vi "Dashboard Main.vi"() -> ()   [LabVIEW 2013]
uses:
  <vilib>/event_ctls.llb/eventvkey.ctl
  <vilib>/Rock Robotics/WPI/Dashboard/WPI_DashboardLogging Global.vi
  <vilib>/Utility/config.llb/Write Key (String).vi
  <vilib>/Utility/config.llb/Write Key (I32).vi
  <vilib>/Utility/config.llb/NI_LVConfig.lvlib
panel:
  out "Image Message":string="Timeout in Camera Communications"
  in  "Rec Mode":enum32{"Stop", "Record", "Playback"}(radio)
  in  "Dashboard Tab":T1(tab)
  in  "Camera Settings":T2={"Frame Rate"=30, "Compression"=30, "Size"=1} {"Frame Rate" scale=1.0..30.0; "Size" items=["640x480", "320x240", "160x120"]}
  out "MotorSliders R":cluster{"MotorSlide1":dbl, "MotorSlide2":dbl} {"MotorSlide2" scale=-1.0..1.0 scale format="%#_2e"; "MotorSlide1" scale=-1.0..1.0 scale format="%#_2e"}
  out "MotorChart R":cluster{"Numeric":dbl, "Numeric":dbl}(graph)
  out "MotorSliders L":T3 {"MotorSlide4 2" scale=0.0..14.0 scale format="%#_2e"; "MotorSlide2" scale=-1.0..1.0 scale format="%#_2e"; "MotorSlide1" scale=-1.0..1.0 scale format="%#_2e"}
  out "MotorChart L":T4(graph)
  out "JS1 Z":dbl(slide) scale=-1.0..1.0 scale format="%#_2e"
  out "Joystick 1":cluster{"X":dbl, "Y":dbl}[](graph)
  out "JS Buttons 1":T5
  out "JS2 Z":dbl(slide) scale=-1.0..1.0 scale format="%#_2e"
  out "Joystick 2":cluster{"X":dbl, "Y":dbl}[](graph)
  out "JS Buttons 2":T5
  out "Mode":T6(ring)=enum."Auto Disabled"
  out "Camera IP":string
  in  "DB Camera Config":bool
  out "fps":dbl format="%#.1g"
  out "Mbps":dbl format="%#.1g"
  out "Mbps 2":bool
  out "LED 1":bool
  in  "Shooter Angle":dbl(slide) scale=20.0..40.0
  out "Averaged Shooter Speed":dbl
  in  "Shooter Speed":dbl(slide) scale=0.0..9.0
  in  "Checkbox 2":bool
  in  "Checkbox 1":bool
  in  "Test Slider":dbl(slide) scale=0.0..100.0 scale format="%#_3g"
  in  "On/Off":bool caption="Solenoid"
  in  "Test Name":u16(ring) items=["Select the test to run...", "Example Test", "-------------------------------", "List of tests is built in robot code.", "Replace with your own automated tests."]
  in  "Test Tree":string(tree)
  in  "Motor":cluster{"Value":dbl, "Enable":bool} {"Value" scale=-1.0..1.0 scale format="%#_3g"}
  out "Progress":T7 {"Test Progress" scale=0.0..100.0}
  in  "Rev/Fwd":cluster{"Forward":bool, "Reverse":bool}
  in  "Test Ring":u16(ring) items=["Auto", "Fixed indoor", "Fixed outdoor 1", "Fixed outdoor 2", "Fixed fluorescent 1", "Fixed fluorescent 2", "Hold current"]
  in  "Listbox":i32(listbox)
  out "Tree":string(tree)
  out "Camera Image":T8(plugin-control)
  in  "Enable":bool
  # "Left"
  # "Front"
  # "Right"
  # "Battery"
  # "This tab is a great place for autonomous settings and validation.\nCustomize by placing controls and indicators here and name to\nmatch Dashboard Variables on robot."
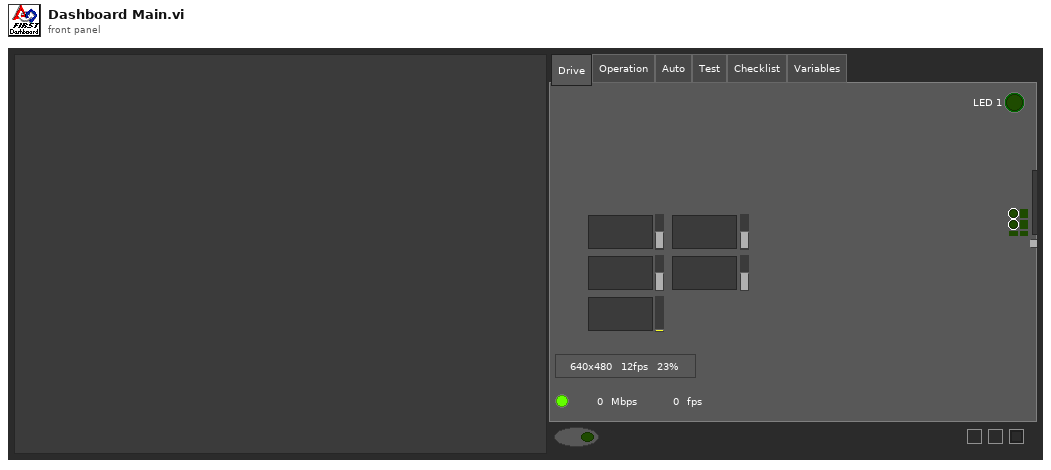
[diagram p1: front panel]
types:
  T1 = enum32{"Drive", "Operation", "Auto", "Test", "Checklist", "Variables"}
  T2 = cluster{"Frame Rate":i32, "Compression":i32, "Size":u16}
  T3 = cluster{"MotorSlide1":dbl, "MotorSlide2":dbl, "MotorSlide4 2":dbl}
  T4 = cluster{"Numeric":dbl, "Numeric":dbl, "Battery":sgl}
  T5 = cluster{bool, bool, bool, bool, bool, bool, bool, bool, bool, bool, bool, bool}
  T6 = enum8{"Tele-Op Disabled", "Tele-Op Enabled", "Auto Disabled", "Auto Enabled", "Test Disabled", "Test Enabled", ""}
  T7 = cluster{"Test Progress":u8, "Test Progress Text":string}
  T8 = typedef "IMAQ Image.ctl" = refnum<image>
  T9 = typedef "Image Type" = u32
  T10 = cluster{"Digital Inputs":bool[], "Digital Outputs":bool[]}
  T11 = cluster{"Competition mode":bool, "Robot Link":bool, "Autonomous":bool, "Enabled":bool, "E-Stop":bool, "Simulated":bool, "TestMode":bool, "Docked Window":bool}
  T12 = cluster{"Boolean Array[0]":bool, "Boolean Array[1]":bool, "Boolean Array[2]":bool, "Boolean Array[3]":bool, "Boolean Array[4]":bool, "Boolean Array[5]":bool, "Boolean Array[6]":bool, "Boolean Array[7]":bool, "Boolean Array[8]":bool, "Boolean Array[9]":bool, "Boolean Array[10]":bool, "Boolean Array[11]":bool}
  T13 = typedef "NI_LVConfig.lvlib/Config Data RefNum.ctl" = refnum<k1>
  T14 = typedef "eventvkey.ctl" = enum16{"ASCII", "Enter", "Return", "Shift", "Ctrl", "Alt", "Cmd", "Opt", "Caps", "NumLock", "Clear", "Break", "Up", "Down", "Left", "Right", "Insert", "Delete", "Home", "End", "PageUp", "PageDown", "Escape", "Help", "Pause", "ScrollLock", "F1", "F2", "F3", "F4", "F5", "F6", "F7", "F8", "F9", "F10", "F11", "F12", "F13", "F14", "F15", "F16", "F17", "F18", "F19", "F20", "F21", "F22", "F23", "F24", "Play", "VolumeUp", "VolumeDown", "Mute", "Two Byte Char"}
  T15 = cluster{"Image Size":bool, "Image Type":bool, "Pixel Value":bool, "ROI Information":bool, "Zoom Factor":bool}
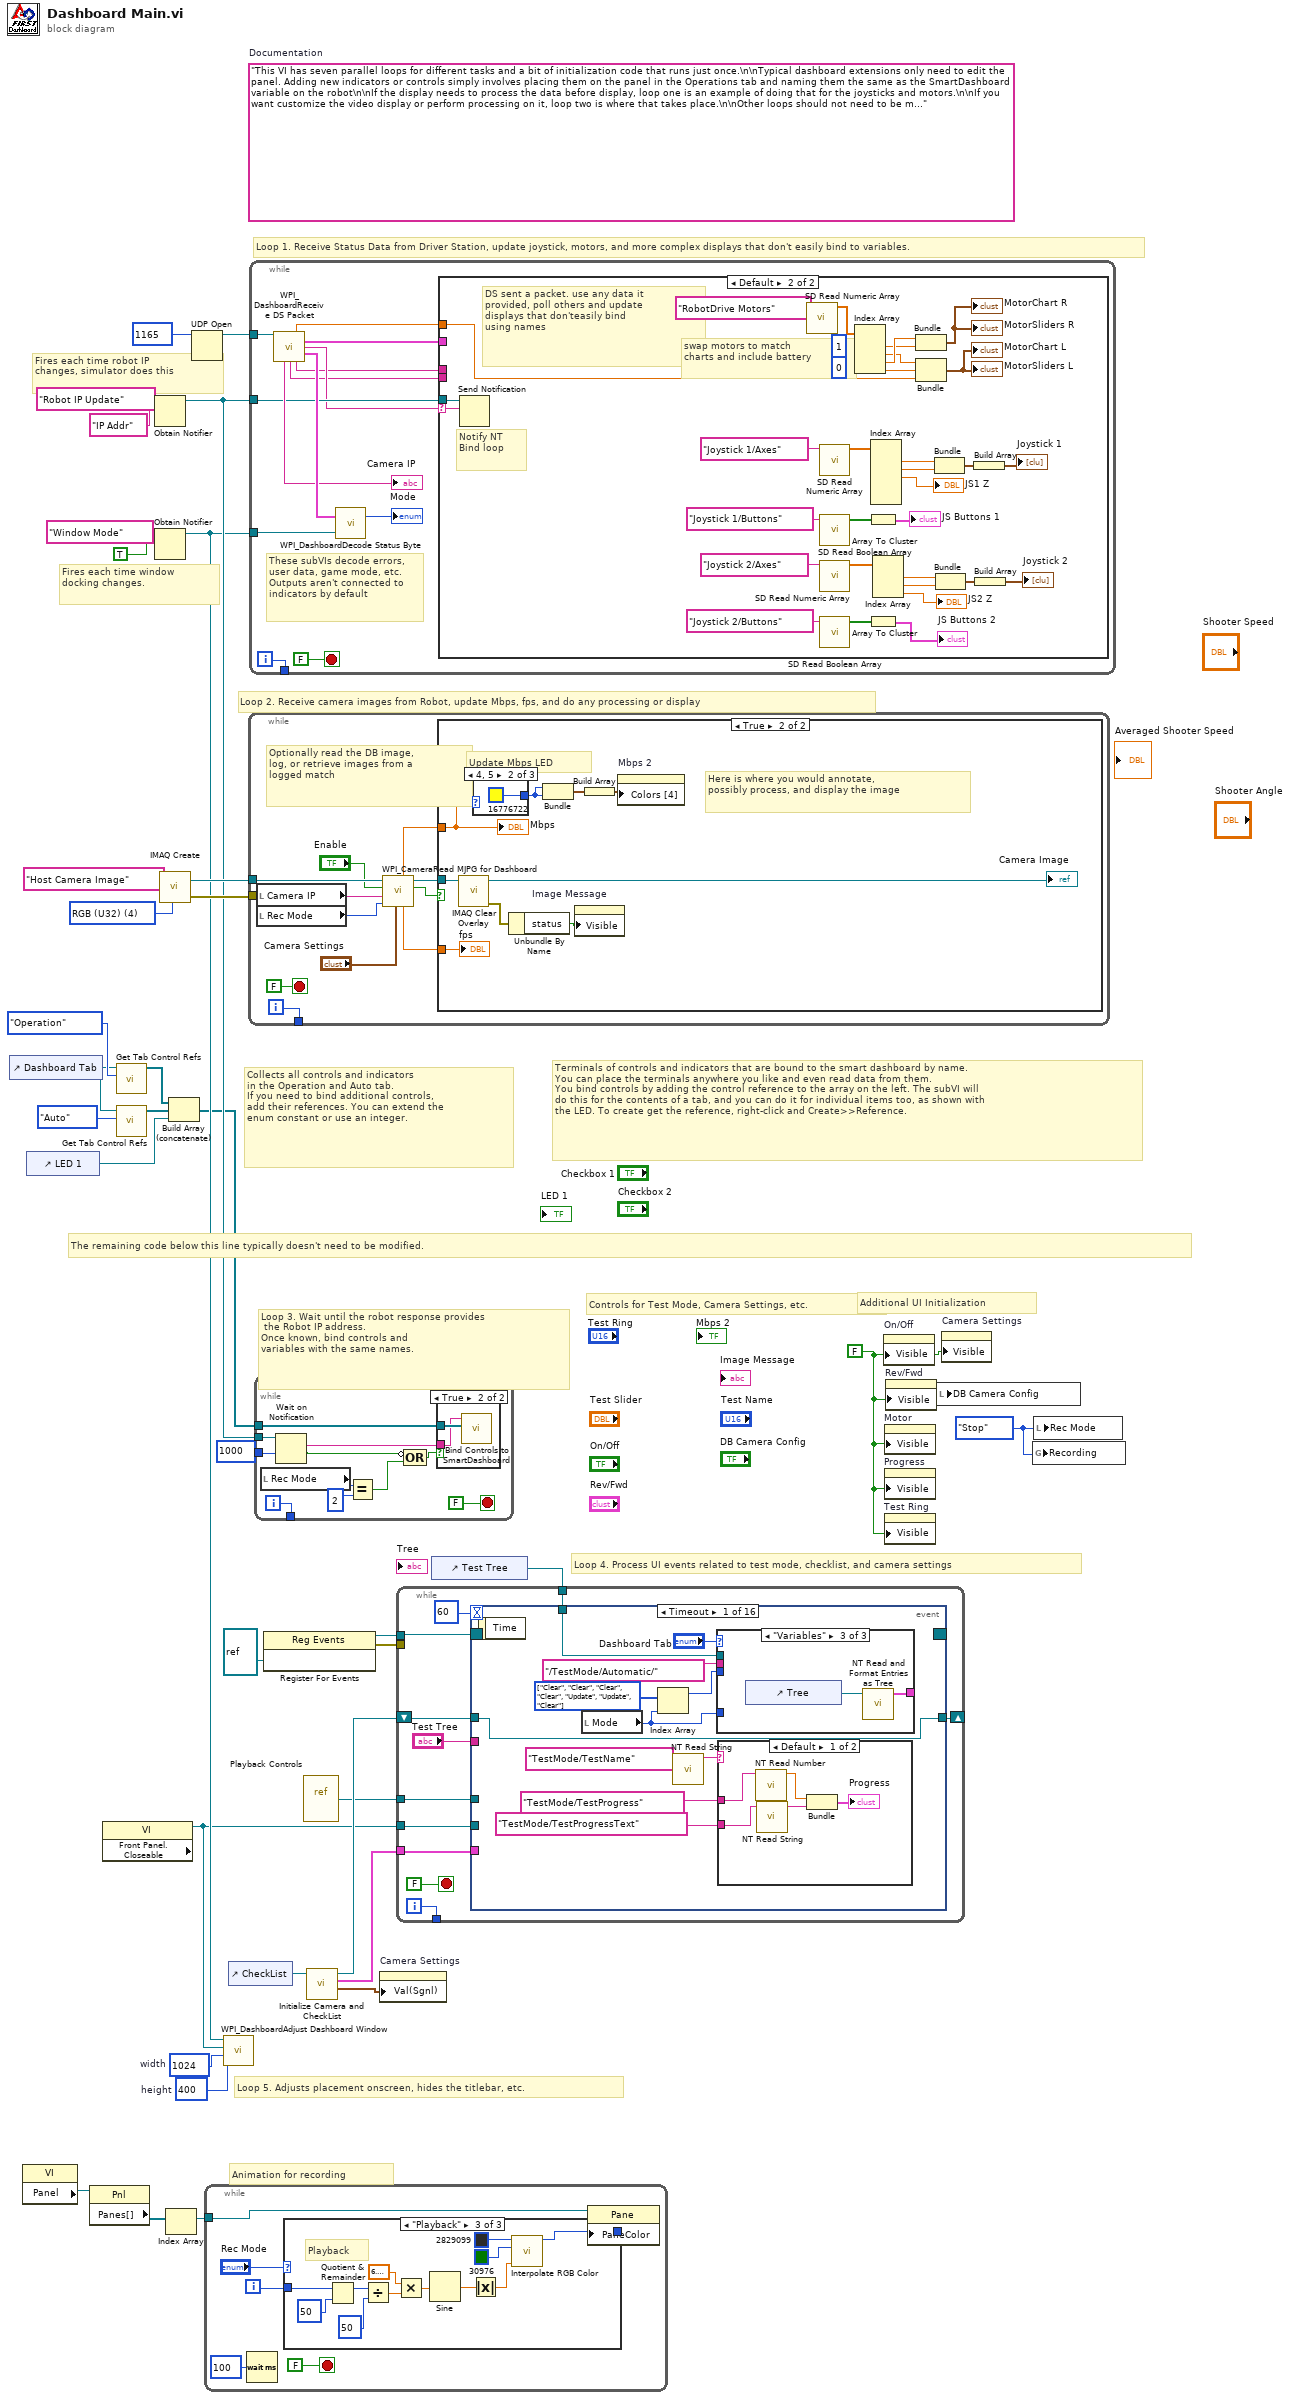
[diagram p0: block diagram]
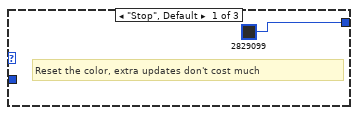
[diagram p2: hidden frame]
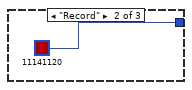
[diagram p3: hidden frame]
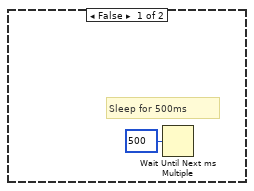
[diagram p5: hidden frame]
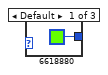
[diagram p6: hidden frame]
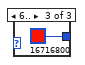
[diagram p7: hidden frame]
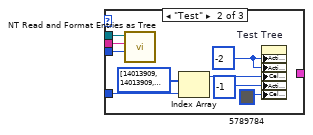
[diagram p9: hidden frame]
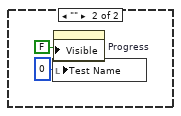
[diagram p10: hidden frame]
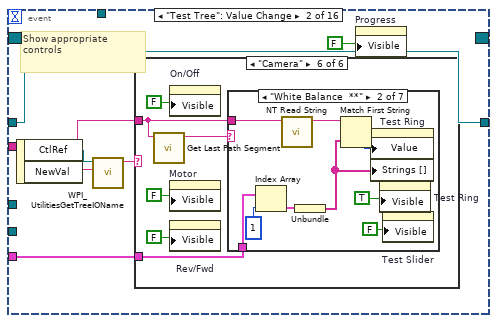
[diagram p11: hidden frame]
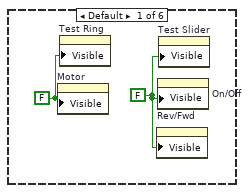
[diagram p12: hidden frame]
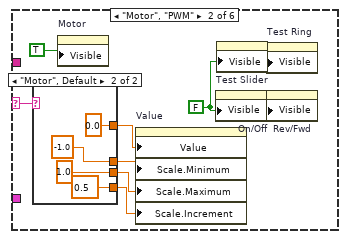
[diagram p13: hidden frame]
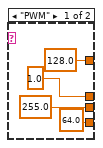
[diagram p14: hidden frame]
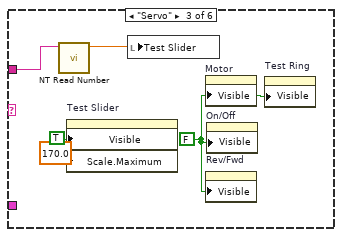
[diagram p15: hidden frame]
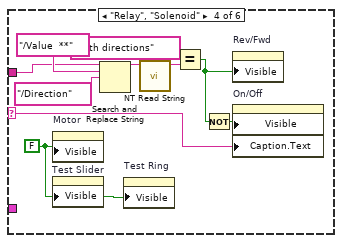
[diagram p16: hidden frame]
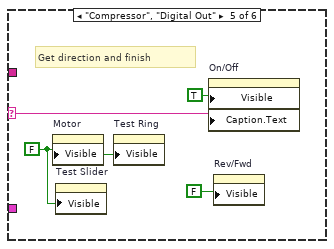
[diagram p17: hidden frame]
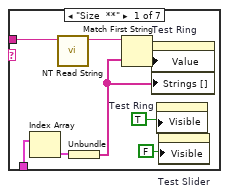
[diagram p18: hidden frame]
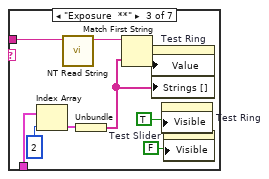
[diagram p19: hidden frame]
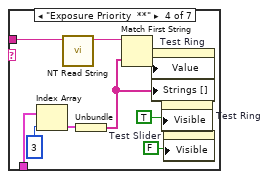
[diagram p20: hidden frame]
diagram:
  w8 = enum32{"Stop", "Record", "Playback"}."Stop" ("Rec Mode")
  w11 = 400  # height
  w12 = 1024  # width
  w25 = FALSE ("Visible")
  (unwired) "This VI has seven parallel loops for different tasks and a bit of initialization code that runs just once.\n\nTypical dashboard extensions only need to edit the panel. Adding new indicators or controls simply involves placing them on the panel in the Operations tab and naming them the same as the SmartDashboard variable on the robot\n\nIf the display needs to process the data before display, loop one is an example of doing that for the joysticks and motors.\n\nIf you want customize the video display or perform processing on it, loop two is where that takes place.\n\nOther loops should not need to be modified. They are pretty standard, and document the task they perform."  # Documentation
  w35 = T9 4 items=["Grayscale (U8)", "Grayscale (I16)", "Grayscale (SGL)", "Complex (CSG)", "RGB (U32)", "HSL (U32)", "RGB (U64)"] ("Image Type")
  # "Controls for Test Mode, Camera Settings, etc."
  # "Additional UI Initialization"
  # "Animation for recording"
  # "Fires each time robot IP\nchanges, simulator does this"
  # "Fires each time window\ndocking changes."
  # "Collects all controls and indicators\nin the Operation and Auto tab.\nIf you need to bind additional controls,\nadd their references. You can extend the\nenum constant or use an integer."
  # "The remaining code below this line typically doesn't need to be modified."
  # "Loop 4. Process UI events related to test mode, checklist, and camera settings"
  # "Terminals of controls and indicators that are bound to the smart dashboard by name.\nYou can place the terminals anywhere you like and even read data from them.\nYou bind controls by adding the control reference to the array on the left. The subVI will\ndo this for the contents of a tab, and you can do it for individual items too, as shown with\nthe LED. To create get the reference, right-click and Create>>Reference."
  # "Loop 3. Wait until the robot response provides\n the Robot IP address.\nOnce known, bind controls and\nvariables with the same names."
  # "Loop 5. Adjusts placement onscreen, hides the titlebar, etc."
  # "Loop 1. Receive Status Data from Driver Station, update joystick, motors, and more complex displays that don't easily bind to variables."
  # "Loop 2. Receive camera images from Robot, update Mbps, fps, and do any processing or display"
  n1 = control-ref of="Dashboard Tab"() -> (w6:refnum<vi>)
  n2 = property class="VI"() -> ("Panel"=w19:refnum<vi>)  [unwired: 2 in, 2 out]
  n3 = control-ref of="LED 1"() -> (w1:refnum<vi>)
  n4 = property class="Pnl"(reference=w19) -> ("Panes[]"=w20:refnum<vi>[])  [unwired: 1 in, 2 out]
  n5 = property class="VI" props=["Front Panel.Closeable"]() -> (reference out=w7:refnum<vi>)  [unwired: 2 in, 2 out]
  n6 = call <vilib>:"Get Tab Control Refs.vi"("Page Index"=T1."Operation" ("Dashboard Tab"), "TabControl in"=w6) -> ("ControlsOnPage"=w4:refnum<vi>[])  [unwired: 9 in]
  n7 = call <vilib>:"Get Tab Control Refs.vi"("Page Index"=T1."Auto" ("Dashboard Tab"), "TabControl in"=w6) -> ("ControlsOnPage"=w5:refnum<vi>[])  [unwired: 9 in]
  n8 = Obtain Notifier(name (unnamed)="Robot IP Update", notification data type="IP Addr" ("name (unnamed)")) -> (notifier out=w29:refnum<notifier>)  [unwired: 2 in, 2 out]
  n9 = Obtain Notifier(name (unnamed)="Window Mode", notification data type=TRUE) -> (notifier out=w10:refnum<notifier>)  [unwired: 2 in, 2 out]
  n10 = call "IMAQ Create"("Image Name"="Host Camera Image", "Image Type"=w35) -> ("New Image"=w33:T8, "error out"=w32:errorcluster)  [unwired: 2 in, 1 out]
  n11 = Index Array(array=w20) -> (element=w18:refnum<vi>)  [unwired: 1 in]
  n12 = Build Array (concatenate)(w4, w5, w1) -> (w3:refnum<vi>[])
  n13 = UDP Open(11:u16 1165 ("port")) -> (port=w36:refnum<k16>)  [unwired: 2 in, 4 out]
  n14 = while {
    tunnel: w18 -> [w39]
    i -> [w42]
    stop <- FALSE stop-if-true
    n15 = Wait (ms)(milliseconds to wait=u32 100) -> ()  [unwired: 1 out]
    n16 = case shown="\"Playback\"" "Rec Mode" {
      tunnel: w42 -> [_ _ w57]
      tunnel: [u32 2829099 ("Base Color") u32 11141120 ("Target Color") w46] -> w38
      frame "Stop", Default {
        # "Reset the color, extra updates don't cost much"
      }
      frame "Record" {
      }
      frame "Playback" {
        # "Playback"
        n17 = Quotient & Remainder(x=w57, y=u32 50 ("milliseconds to wait")) -> (x-y*floor(x/y)=w53:u32)  [unwired: 1 out]
        n18 = Divide(x=w53, y=u32 50 ("milliseconds to wait")) -> (x/y=w50:dbl)
        n19 = Multiply(x=6.283185307179586, y=w50) -> (x*y=w55:dbl)
        n20 = Sine(x=w55) -> (sin(x)=w54:dbl)
        n21 = Absolute Value(x=w54) -> (abs(x)=w47:dbl)
        n22 = call "Interpolate RGB Color.vi"("Proportion"=w47, "Target Color"=u32 30976, "Base Color"=u32 2829099) -> ("Result Color"=w46:u32)  [unwired: 8 in]
      }
    }
    n23 = property class="Pane"(reference=w39, "PaneColor"=w38) -> ()  [unwired: 1 in, 2 out]
  }
  n24 = call <vilib>:"WPI_DashboardAdjust Dashboard Window.vi"("height"=w11, "width"=w12, "reference in"=w7, "Notifier in"=w10) -> ()  [unwired: 8 in]
  n25 = control-ref of="CheckList"() -> (w9:refnum<vi>)
  n26 = while {
    tunnel: w33 -> [w66]
    tunnel: w32 -> [_]
    tunnel: [w67] -> _
    i -> [w67]
    stop <- FALSE stop-if-true
    # "Optionally read the DB image,\nlog, or retrieve images from a\nlogged match"
    n27 = local read "Camera IP"() -> (w59:string)
    n28 = local read "Rec Mode"() -> (w58:enum32{"Stop", "Record", "Playback"})
    n29 = call <vilib>:"WPI_CameraRead MJPG for Dashboard.vi"("Camera Settings"="Camera Settings", "Rec Mode"=w58, "Camera IP"=w59, "Enable"="Enable", "Refnum in"=w66) -> ("Active"=w63:bool, "Refnum out"=w65:T8, "FPS"=w62:dbl, "Bandwidth (Mbps)"=w61:dbl)  [unwired: 3 in]
    n30 = case shown="True" w63 {
      tunnel: w65 -> [_ w73]
      tunnel: w61 -> [_ w72]
      tunnel: w62 -> [_ w70]
      frame False {
        # "Sleep for 500ms"
        n31 = Wait Until Next ms Multiple(millisecond multiple=u32 500) -> ()  [unwired: 1 out]
      }
      frame True {
        # "Here is where you would annotate,\npossibly process, and display the image"
        # "Update Mbps LED"
        n32 = call "IMAQ Clear Overlay"("Image"=w73) -> ("error out"=w77:errorcluster, "Image Out"=→"Camera Image":T8)  [unwired: 2 in, 7 out]
        n33 = case shown="4, 5" w72 {
          tunnel: [u32 6618880 ("Color Box") u32 16776722 ("Color Box") u32 16716800 ("Color Box")] -> w74
          frame Default {
          }
          frame 4, 5 {
          }
          frame 6.. {
          }
        }
        n34 = Unbundle By Name(w77) -> ("status"=w78:bool)
        n35 = Bundle("Color Box"=w74, "Color Box"=w74) -> (w76:cluster{"Color Box":u32, "Color Box":u32})  [unwired: 1 out]
        n36 = property on="Image Message" class="Str"("Visible"=w78) -> ()  [unwired: 2 in, 2 out]
        n37 = Build Array(w76) -> (w75:cluster{"Color Box":u32, "Color Box":u32}[])
        n38 = property on="Mbps 2" class="Bool (strict)"("Colors [4]"=w75) -> ()  [unwired: 2 in, 2 out]
        "Mbps" <- w72
        "fps" <- w70
      }
    }
  }
  n39 = while {
    tunnel: w36 -> [w92]
    tunnel: w29 -> [w87]
    tunnel: w10 -> [w91]
    tunnel: [w88] -> _
    i -> [w88]
    stop <- FALSE stop-if-true
    # "These subVIs decode errors, user data, game mode, etc.\nOutputs aren't connected to indicators by default"
    n40 = call <vilib>:"WPI_DashboardReceive DS Packet.vi"("Recv Socket"=w92) -> ("Battery"=w82:sgl, "Driver Station"=w83:T10, "Robot IP Address"=w86:string, "Status"=w93:T11, "Camera IP Address"=→"Camera IP":string, "Low Priority User Data"=w85:string, "High Priority User Data"=w84:string)  [unwired: 1 in, 7 out]
    n41 = call <vilib>:"WPI_DashboardDecode Status Byte.vi"("Window Mode Notifier"=w91, "Status"=w93) -> ("Mode"=→"Mode":T6)  [unwired: 1 out]
    n42 = case shown="Default" w86 {
      selector: w86 -> [_ w105]
      tunnel: w87 -> [_ w106]
      tunnel: w85 -> [_ _]
      tunnel: w84 -> [_ _]
      tunnel: w83 -> [_ _]
      tunnel: w82 -> [_ w104]
      frame "0.0.0.0" {
        # "DS not sending packets, or no robot exists yet.\nDon't poll the variables"
      }
      frame Default {
        # "Notify NT\nBind loop"
        # "DS sent a packet. use any data it\nprovided, poll others and update\ndisplays that don'teasily bind\nusing names"
        # "swap motors to match\ncharts and include battery"
        n43 = Send Notification(notification=w105, notifier=w106) -> ()  [unwired: 1 in, 2 out]
        n44 = call <vilib>:"SD Read Numeric Array.vi"("Name"="RobotDrive Motors") -> ("Numeric Array"=w103:dbl[])  [unwired: 8 in, 2 out]
        n45 = call <vilib>:"SD Read Numeric Array.vi"("Name"="Joystick 1/Axes") -> ("Numeric Array"=w122:dbl[])  [unwired: 8 in, 2 out]
        n46 = call <vilib>:"SD Read Boolean Array.vi"("Name"="Joystick 1/Buttons") -> ("Boolean Array"=w124:bool[])  [unwired: 8 in, 2 out]
        n47 = call <vilib>:"SD Read Numeric Array.vi"("Name"="Joystick 2/Axes") -> ("Numeric Array"=w116:dbl[])  [unwired: 8 in, 2 out]
        n48 = call <vilib>:"SD Read Boolean Array.vi"("Name"="Joystick 2/Buttons") -> ("Boolean Array"=w115:bool[])  [unwired: 8 in, 2 out]
        n49 = Index Array(array=w103, index #1=1, index #4=0) -> (element #1=w99:dbl, element #2=w98:dbl, element #3=w100:dbl, element #4=w95:dbl)  [unwired: 2 in]
        n50 = Array To Cluster(array=w124) -> (cluster=→"JS Buttons 1":T12)
        n51 = Array To Cluster(array=w115) -> (cluster=→"JS Buttons 2":T12)
        n52 = Index Array(array=w122) -> (element #1=w119:dbl, element #2=w120:dbl, element #3=→"JS1 Z":dbl)  [unwired: 6 in, 3 out]
        n53 = Index Array(array=w116) -> (element #1=w111:dbl, element #2=w110:dbl, element #3=→"JS2 Z":dbl)  [unwired: 3 in]
        n54 = Bundle("Numeric"=w100, "Numeric"=w99) -> (→"MotorChart R" →"MotorSliders R":cluster{"Numeric":dbl, "Numeric":dbl})  [unwired: 1 in]
        n55 = Bundle("Numeric"=w98, "Numeric"=w95, "Battery"=w104) -> (→"MotorChart L" →"MotorSliders L":T4)  [unwired: 1 in]
        n56 = Bundle("Numeric"=w119, "Numeric"=w120) -> (w118:cluster{"Numeric":dbl, "Numeric":dbl})  [unwired: 1 in]
        n57 = Bundle("Numeric"=w111, "Numeric"=w110) -> (w112:cluster{"Numeric":dbl, "Numeric":dbl})  [unwired: 1 in]
        n58 = Build Array(w118) -> (→"Joystick 1":cluster{"Numeric":dbl, "Numeric":dbl}[])
        n59 = Build Array(w112) -> (→"Joystick 2":cluster{"Numeric":dbl, "Numeric":dbl}[])
      }
    }
  }
  n60 = while {
    tunnel: w3 -> [w138]
    tunnel: w29 -> [w136]
    tunnel: [w134] -> _
    tunnel: u32 1000 ("milliseconds to wait") -> [w133]
    i -> [w134]
    stop <- FALSE stop-if-true
    n61 = local read "Rec Mode"() -> (w129:enum32{"Stop", "Record", "Playback"})
    n62 = Wait on Notification(notifier=w136, timeout in ms (-1)=w133) -> (notification=w135:string, timed out?=w131:bool)  [unwired: 2 in, 2 out]
    n63 = Equal?(x=w129, y=u16 2 ("Rec Mode")) -> (x = y?=w130:bool)
    n64 = Compound Arithmetic op=OR(invert w131, w130) -> (w132:bool)
    n65 = case shown="True" w132 {
      tunnel: w138 -> [_ w140]
      tunnel: w135 -> [_ w139]
      frame False {
      }
      frame True {
        n66 = call <vilib>:"Bind Controls to SmartDashboard.vi"("Bound Control Refs"=w140, "Server IP Address"=w139) -> ()  [unwired: 10 in]
      }
    }
  }
  n67 = register-events(refnum<vi> refnum) -> (reference out=w16:refnum<event-registration>, error out=w15:errorcluster)  [unwired: 2 in]
  n68 = vi-ref "Playback Controls.vi"() -> (w17:refnum<vi>)
  n69 = call "Initialize Camera and CheckList.vi"("ListBox in"=w9) -> ("Cluster"=w23:cluster{"value":i32, "value":i32, "index":i32}, "Array"=w24:cluster{string[]}[], "File Refnum"=w22:T13)  [unwired: 8 in]
  n70 = property on="Camera Settings" class="Clust (strict)"("Val(Sgnl)"=w23) -> ()  [unwired: 2 in, 2 out]
  n71 = control-ref of="Test Tree"() -> (w21:refnum<vi>)
  n72 = while {
    tunnel: w24 -> [w148]
    shift-right: [w147] -> _
    shift-left: w22 -> [w146]
    tunnel: [w145] -> _
    tunnel: w21 -> [w144]
    tunnel: w17 -> [w143]
    tunnel: w16 -> [w142]
    tunnel: w15 -> [_]
    tunnel: w7 -> [w141]
    i -> [w145]
    stop <- FALSE stop-if-true
    n73 = event shown="[0] Timeout" {
      selector: w142 -> [_ _ _ _ _ _ _ _ _ _ _ _ _ _ _ _]
      dyn-events: [_ _ _ _ _ _ _ _ _ _ _ _ _ w386 _ _] -> _
      timeout: u32 60 ("milliseconds to wait") -> [_ _ _ _ _ _ _ _ _ _ _ _ _ _ _ _]
      tunnel: w144 -> [w158 _ _ _ _ _ _ _ _ _ _ _ _ _ _ _]
      tunnel: "Test Tree" -> [_ _ _ _ _ _ _ _ w355 w363 w365 w369 w377 _ _ _]
      tunnel: w148 -> [_ w182 _ _ _ _ w319 w349 _ _ _ _ _ _ _ _]
      tunnel: [w152 w181 w280 w285 w293 w305 w318 w342 w354 w361 w364 w368 w376 w388 w402 w403] -> w147
      tunnel: w146 -> [w152 w181 w280 w285 w293 w305 w317 w342 w354 w361 w364 w368 w376 w388 w402 w403]
      tunnel: w143 -> [_ _ _ _ _ _ _ _ _ _ _ _ _ w389 _ w406]
      tunnel: w141 -> [_ _ _ _ _ _ _ _ _ _ _ _ _ w384 _ _]
      event Timeout {
        w157 = enum16{"Update", "Clear"}[] [enum."Clear", enum."Clear", enum."Clear", enum."Clear", enum."Update", enum."Update", enum."Clear"] items=["Update", "Clear"]
        n74 = event-data() -> ()  [unwired: 1 in, 1 out]
        n75 = local read "Mode"() -> (w155:T6)
        n76 = Index Array(array=w157, index=w155) -> (element=w156:enum16{"Update", "Clear"})
        n77 = call <vilib>:"NT Read String.vi"("Name"="TestMode/TestName") -> ("String"=w161:string)  [unwired: 9 in, 1 out]
        n78 = case shown="\"Variables\"" "Dashboard Tab" {
          tunnel: w158 -> [_ w171 _]
          tunnel: "/TestMode/Automatic/" ("Name Pattern") -> [_ w170 _]
          tunnel: w156 -> [_ w169 _]
          tunnel: w155 -> [_ w167 _]
          tunnel: [_ _ w173] -> _
          frame "Operation", Default {
          }
          frame "Test" {
            w166 = -2 ("Active Item:Row Number")
            n79 = call <vilib>:"NT Read and Format Entries as Tree.vi"("Operation"=w169, "Name Pattern"=w170, "Tree Refnum"=w171) -> ()  [unwired: 7 in, 2 out]
            n80 = Index Array(array=u32[] [14013909, 14013909, 14013909, 14013909, 14013909, 16777215, 14013909], index=w167) -> (element=w165:u32)
            n81 = property on="Test Tree" class="Tree (strict)"("Active Item Row Number"=w166, "ActiveColNum"=w166, "CellBG"=w165, "Active Item Row Number"=-1 ("Active Item:Row Number"), "CellBG"=u32 5789784 ("Color Box")) -> ()  [unwired: 2 in, 2 out]
          }
          frame "Variables" {
            n82 = control-ref of="Tree"() -> (w172:refnum<vi>)
            n83 = call <vilib>:"NT Read and Format Entries as Tree.vi"("Tree Refnum"=w172) -> ("Formatted Strings"=w173:cluster{"Name":string, "Value":string}[])  [unwired: 9 in, 1 out]
          }
        }
        n84 = case shown="Default" w161 {
          tunnel: "TestMode/TestProgress" ("Name") -> [w175 _]
          tunnel: "TestMode/TestProgressText" ("Name") -> [w174 _]
          frame Default {
            n85 = call <vilib>:"NT Read Number.vi"("Name"=w175) -> ("Numeric"=w176:dbl)  [unwired: 9 in, 1 out]
            n86 = call <vilib>:"NT Read String.vi"("Name"=w174) -> ("String"=w177:string)  [unwired: 9 in, 1 out]
            n87 = Bundle("Numeric"=w176, "String"=w177) -> (→"Progress":cluster{"Numeric":dbl, "String":string})  [unwired: 1 in]
          }
          frame "" {
            n88 = local write "Test Name"(u16 0) -> ()
            n89 = property on="Progress" class="Clust (strict)"("Visible"=FALSE) -> ()  [unwired: 2 in, 2 out]
          }
        }
      }
      event "Test Tree": Value Change {
        # "Show appropriate\ncontrols"
        n90 = event-data() -> ("CtlRef"=w185:refnum<vi>, "NewVal"=w183:string)  [unwired: 1 in]
        n91 = call <vilib>:"WPI_UtilitiesGetTreeIOName.vi"("NewVal"=w183, "TreeControl in"=w185) -> ("I/O Name"=w186:string)  [unwired: 9 in]
        n92 = case shown="\"Camera\"" w186 {
          selector: w186 -> [_ w193 _ w211 w220 _]
          tunnel: w183 -> [_ _ w208 w210 _ w227]
          tunnel: w182 -> [_ _ _ _ _ w226]
          frame Default {
            w188 = FALSE ("Visible")
            w187 = FALSE ("Visible")
            n93 = property on="Motor" class="Clust (strict)"("Visible"=w187) -> ()  [unwired: 2 in, 2 out]
            n94 = property on="Test Ring" class="Ring (strict)"("Visible"=w187) -> ()  [unwired: 2 in, 2 out]
            n95 = property on="Rev/Fwd" class="Clust (strict)"("Visible"=w188) -> ()  [unwired: 2 in, 2 out]
            n96 = property on="On/Off" class="Bool (strict)"("Visible"=w188) -> ()  [unwired: 2 in, 2 out]
            n97 = property on="Test Slider" class="Slide (strict)"("Visible"=w188) -> ()  [unwired: 2 in, 2 out]
          }
          frame "Motor", "PWM" {
            w194 = FALSE ("Visible")
            n98 = case shown="\"Motor\", Default" w193 {
              tunnel: [1.0 ("Value") -1.0 ("Value")] -> w192
              tunnel: [255.0 ("Value") 1.0 ("Value")] -> w191
              tunnel: [128.0 ("Value") 0.0 ("Value")] -> w190
              tunnel: [64.0 ("Value") 0.5 ("Value")] -> w189
              frame "PWM" {
              }
              frame "Motor", Default {
              }
            }
            n99 = property on="Motor" class="Clust (strict)"("Visible"=TRUE) -> ()  [unwired: 2 in, 2 out]
            n100 = property on="Value" class="Slide (strict)"("Value"=w190, "Scale.Minimum"=w192, "Scale.Maximum"=w191, "Scale.Increment"=w189) -> ()  [unwired: 2 in, 2 out]
            n101 = property on="On/Off" class="Bool (strict)"("Visible"=w194) -> ()  [unwired: 2 in, 2 out]
            n102 = property on="Test Slider" class="Slide (strict)"("Visible"=w194) -> ()  [unwired: 2 in, 2 out]
            n103 = property on="Test Ring" class="Ring (strict)"("Visible"=w194) -> ()  [unwired: 2 in, 2 out]
            n104 = property on="Rev/Fwd" class="Clust (strict)"("Visible"=w194) -> ()  [unwired: 2 in, 2 out]
          }
          frame "Servo" {
            w206 = FALSE ("Visible")
            n105 = call <vilib>:"NT Read Number.vi"("Name"=w208) -> ("Numeric"=w207:dbl)  [unwired: 9 in, 1 out]
            n106 = property on="Test Slider" class="Slide (strict)"("Visible"=TRUE, "Scale.Maximum"=170.0 ("Scale.Range:Maximum")) -> ()  [unwired: 2 in, 2 out]
            n107 = local write "Test Slider"(w207) -> ()
            n108 = property on="Motor" class="Clust (strict)"("Visible"=w206) -> ()  [unwired: 2 in, 2 out]
            n109 = property on="Rev/Fwd" class="Clust (strict)"("Visible"=w206) -> ()  [unwired: 2 in, 2 out]
            n110 = property on="On/Off" class="Bool (strict)"("Visible"=w206) -> ()  [unwired: 2 in, 2 out]
            n111 = property on="Test Ring" class="Ring (strict)"("Visible"=w206) -> ()  [unwired: 2 in, 2 out]
          }
          frame "Relay", "Solenoid" {
            w209 = FALSE ("Visible")
            n112 = property on="Motor" class="Clust (strict)"("Visible"=w209) -> ()  [unwired: 2 in, 2 out]
            n113 = property on="Test Slider" class="Slide (strict)"("Visible"=w209) -> ()  [unwired: 2 in, 2 out]
            n114 = Search and Replace String(input string=w210, search string="/Value  **", replace string="/Direction") -> (result string=w216:string)  [unwired: 5 in, 3 out]
            n115 = property on="Test Ring" class="Ring (strict)"("Visible"=w209) -> ()  [unwired: 2 in, 2 out]
            n116 = call <vilib>:"NT Read String.vi"("Name"=w216) -> ("String"=w214:string)  [unwired: 9 in, 1 out]
            n117 = Equal?(x="Both directions", y=w214) -> (x = y?=w212:bool)
            n118 = Not(x=w212) -> (.not. x?=w213:bool)
            n119 = property on="Rev/Fwd" class="Clust (strict)"("Visible"=w212) -> ()  [unwired: 2 in, 2 out]
            n120 = property on="On/Off" class="Bool (strict)"("Visible"=w213, "Caption.Text"=w211) -> ()  [unwired: 2 in, 2 out]
          }
          frame "Compressor", "Digital Out" {
            w219 = FALSE ("Visible")
            # "Get direction and finish"
            n121 = property on="Motor" class="Clust (strict)"("Visible"=w219) -> ()  [unwired: 2 in, 2 out]
            n122 = property on="Test Slider" class="Slide (strict)"("Visible"=w219) -> ()  [unwired: 2 in, 2 out]
            n123 = property on="Test Ring" class="Ring (strict)"("Visible"=w219) -> ()  [unwired: 2 in, 2 out]
            n124 = property on="On/Off" class="Bool (strict)"("Visible"=TRUE, "Caption.Text"=w220) -> ()  [unwired: 2 in, 2 out]
            n125 = property on="Rev/Fwd" class="Clust (strict)"("Visible"=FALSE) -> ()  [unwired: 2 in, 2 out]
          }
          frame "Camera" {
            n126 = call <vilib>:"Get Last Path Segment.vi"("String in"=w227) -> ("String out"=w228:string)  [unwired: 10 in]
            n127 = property on="On/Off" class="Bool (strict)"("Visible"=FALSE) -> ()  [unwired: 2 in, 2 out]
            n128 = property on="Motor" class="Clust (strict)"("Visible"=FALSE) -> ()  [unwired: 2 in, 2 out]
            n129 = property on="Rev/Fwd" class="Clust (strict)"("Visible"=FALSE) -> ()  [unwired: 2 in, 2 out]
            n130 = case shown="\"White Balance  **\"" w228 {
              tunnel: w227 -> [w234 w243 w252 w261 w270 _ w276]
              tunnel: w226 -> [w232 w240 w249 w258 w267 _ _]
              frame "Size  **" {
                n131 = Index Array(array=w232) -> (element=w231:cluster{string[]})  [unwired: 1 in]
                n132 = call <vilib>:"NT Read String.vi"("Name"=w234) -> ("String"=w233:string)  [unwired: 9 in, 1 out]
                n133 = Unbundle(w231) -> (w229:string[])
                n134 = Match First String(2:w229, 3:w233) -> (0:w230:i32)  [unwired: 1 out]
                n135 = property on="Test Ring" class="Ring (strict)"("Value"=w230, "Strings []"=w229) -> ()  [unwired: 2 in, 2 out]
                n136 = property on="Test Ring" class="Ring (strict)"("Visible"=TRUE) -> ()  [unwired: 2 in, 2 out]
                n137 = property on="Test Slider" class="Slide (strict)"("Visible"=FALSE) -> ()  [unwired: 2 in, 2 out]
              }
              frame "White Balance  **" {
                n138 = Index Array(array=w240, index=1) -> (element=w241:cluster{string[]})
                n139 = call <vilib>:"NT Read String.vi"("Name"=w243) -> ("String"=w242:string)  [unwired: 9 in, 1 out]
                n140 = Unbundle(w241) -> (w238:string[])
                n141 = Match First String(2:w238, 3:w242) -> (0:w237:i32)  [unwired: 1 out]
                n142 = property on="Test Ring" class="Ring (strict)"("Value"=w237, "Strings []"=w238) -> ()  [unwired: 2 in, 2 out]
                n143 = property on="Test Ring" class="Ring (strict)"("Visible"=TRUE) -> ()  [unwired: 2 in, 2 out]
                n144 = property on="Test Slider" class="Slide (strict)"("Visible"=FALSE) -> ()  [unwired: 2 in, 2 out]
              }
              frame "Exposure  **" {
                n145 = Index Array(array=w249, index=2) -> (element=w250:cluster{string[]})
                n146 = call <vilib>:"NT Read String.vi"("Name"=w252) -> ("String"=w251:string)  [unwired: 9 in, 1 out]
                n147 = Unbundle(w250) -> (w246:string[])
                n148 = Match First String(2:w246, 3:w251) -> (0:w247:i32)  [unwired: 1 out]
                n149 = property on="Test Ring" class="Ring (strict)"("Value"=w247, "Strings []"=w246) -> ()  [unwired: 2 in, 2 out]
                n150 = property on="Test Ring" class="Ring (strict)"("Visible"=TRUE) -> ()  [unwired: 2 in, 2 out]
                n151 = property on="Test Slider" class="Slide (strict)"("Visible"=FALSE) -> ()  [unwired: 2 in, 2 out]
              }
              frame "Exposure Priority  **" {
                n152 = Index Array(array=w258, index=3) -> (element=w259:cluster{string[]})
                n153 = call <vilib>:"NT Read String.vi"("Name"=w261) -> ("String"=w260:string)  [unwired: 9 in, 1 out]
                n154 = Unbundle(w259) -> (w255:string[])
                n155 = Match First String(2:w255, 3:w260) -> (0:w256:i32)  [unwired: 1 out]
                n156 = property on="Test Ring" class="Ring (strict)"("Value"=w256, "Strings []"=w255) -> ()  [unwired: 2 in, 2 out]
                n157 = property on="Test Ring" class="Ring (strict)"("Visible"=TRUE) -> ()  [unwired: 2 in, 2 out]
                n158 = property on="Test Slider" class="Slide (strict)"("Visible"=FALSE) -> ()  [unwired: 2 in, 2 out]
              }
              frame "Color Enable  **" {
                n159 = Index Array(array=w267, index=4) -> (element=w268:cluster{string[]})
                n160 = call <vilib>:"NT Read String.vi"("Name"=w270) -> ("String"=w269:string)  [unwired: 9 in, 1 out]
                n161 = Unbundle(w268) -> (w264:string[])
                n162 = Match First String(2:w264, 3:w269) -> (0:w265:i32)  [unwired: 1 out]
                n163 = property on="Test Ring" class="Ring (strict)"("Value"=w265, "Strings []"=w264) -> ()  [unwired: 2 in, 2 out]
                n164 = property on="Test Ring" class="Ring (strict)"("Visible"=TRUE) -> ()  [unwired: 2 in, 2 out]
                n165 = property on="Test Slider" class="Slide (strict)"("Visible"=FALSE) -> ()  [unwired: 2 in, 2 out]
              }
              frame Default {
                n166 = property on="Test Ring" class="Ring (strict)"("Visible"=FALSE) -> ()  [unwired: 2 in, 2 out]
                n167 = property on="Test Slider" class="Slide (strict)"("Visible"=FALSE) -> ()  [unwired: 2 in, 2 out]
              }
              frame "Brightness  **", "Color Level  **", "Compression  **", "FPS  **", "Sharpness  **" {
                n168 = call <vilib>:"NT Read Number.vi"("Name"=w276) -> ("Numeric"=w275:dbl)  [unwired: 9 in, 1 out]
                n169 = local write "Test Slider"(w275) -> ()
                n170 = property on="Test Slider" class="Slide (strict)"("Visible"=TRUE, "Scale.Maximum"=100.0 ("Scale.Range:Maximum")) -> ()  [unwired: 2 in, 2 out]
                n171 = property on="Test Ring" class="Ring (strict)"("Visible"=FALSE) -> ()  [unwired: 2 in, 2 out]
              }
            }
          }
        }
        n172 = property on="Progress" class="Clust (strict)"("Visible"=FALSE) -> ()  [unwired: 2 in, 2 out]
      }
      event "Test Name": Mouse Enter {
        # "Populate the ring with the list of tests"
        n173 = event-data() -> ()  [unwired: 1 in, 1 out]
        n174 = call <vilib>:"NT Read String Array.vi"("Name"="TestMode/TestList") -> ("String Array"=w284:string[])  [unwired: 9 in, 1 out]
        n175 = Build Array (concatenate)("Select the test to run...", w284) -> (w283:string[])
        n176 = property on="Test Name" class="Ring (strict)"("Strings []"=w283) -> ()  [unwired: 2 in, 2 out]
      }
      event "Test Name": Value Change {
        w286 = FALSE ("Visible")
        # "Tell the robot the test name to run"
        n177 = event-data() -> ("NewVal"=w290:u16)  [unwired: 1 in]
        n178 = property on="Test Name" class="Ring (strict)"() -> ("Strings []"=w291:string[])  [unwired: 2 in, 2 out]
        n179 = local write "Progress"(T7 {"Test Progress"=0, "Test Progress Text"=""} ("Progress")) -> ()
        n180 = Index Array(array=w291, index=w290) -> (element=w289:string)
        n181 = call <vilib>:"NT Write String.vi"("String"=w289, "Name"="TestMode/TestName") -> ()  [unwired: 9 in, 1 out]
        n182 = property on="Progress" class="Clust (strict)"("Visible"=TRUE) -> ()  [unwired: 2 in, 2 out]
        n183 = property on="Motor" class="Clust (strict)"("Visible"=w286) -> ()  [unwired: 2 in, 2 out]
        n184 = property on="Test Slider" class="Slide (strict)"("Visible"=w286) -> ()  [unwired: 2 in, 2 out]
        n185 = property on="On/Off" class="Bool (strict)"("Visible"=w286) -> ()  [unwired: 2 in, 2 out]
        n186 = property on="Rev/Fwd" class="Clust (strict)"("Visible"=w286) -> ()  [unwired: 2 in, 2 out]
        n187 = property on="Test Ring" class="Ring (strict)"("Visible"=w286) -> ()  [unwired: 2 in, 2 out]
      }
      event "Listbox": Double Click {
        n188 = event-data() -> ("PlatMods.Shift"=w294:bool, "Row"=w296:i32)  [unwired: 1 in]
        n189 = case shown="True" w294 {
          tunnel: w296 -> [w300 _]
          tunnel: 1 -> [w299 _]
          frame False {
            n190 = property on="Listbox" class="LstBox (strict)"() -> ("Item Symbols"=w298:i32[])  [unwired: 2 in, 2 out]
            n191 = Replace Array Subset(array=w298, new element=w299, index=w300) -> (w297:i32[])
            n192 = property on="Listbox" class="LstBox (strict)"("Item Symbols"=w297) -> ()  [unwired: 2 in, 2 out]
          }
          frame True {
            w301 = 0 ("Top Row")
            n193 = property on="Listbox" class="LstBox (strict)"() -> ("Number of Rows"=w303:u32)  [unwired: 2 in, 2 out]
            n194 = Initialize Array(0, w303) -> (w302:i32[])
            n195 = property on="Listbox" class="LstBox (strict)"("Top Row"=w301, "Value"=w301, "Item Symbols"=w302) -> ()  [unwired: 2 in, 2 out]
          }
        }
      }
      event "Listbox": Key Down {
        n196 = event-data() -> ("VKey"=w307:T14)  [unwired: 1 in]
        n197 = case shown="\"Left\", \"Right\"" w307 {
          selector: w307 -> [w312 _]
          tunnel: eventvkey."Left" ("VKey") -> [w310 _]
          frame "Left", "Right" {
            n198 = Equal?(x=w310, y=w312) -> (x = y?=w311:bool)
            n199 = Select(t=0, s=w311, f=1) -> (s? t:f=w313:i32)
            n200 = property on="Listbox" class="LstBox (strict)"() -> ("Item Symbols"=w316:i32[])  [unwired: 2 in, 2 out]
            n201 = Replace Array Subset(array=w316, new element=w313, index="Listbox") -> (w315:i32[])
            n202 = property on="Listbox" class="LstBox (strict)"("Item Symbols"=w315) -> ()  [unwired: 2 in, 2 out]
          }
          frame Default {
          }
        }
      }
      event "DB Camera Config": Value Change {
        n203 = event-data() -> ("NewVal"=w320:bool)  [unwired: 1 in]
        n204 = case shown="False" w320 {
          tunnel: w319 -> [w329 _]
          tunnel: [w322 w340] -> w318
          tunnel: w317 -> [w321 w340]
          frame False {
            w336 = "Camera"
            w339 = FALSE ("Visible")
            n205 = local read "Camera Settings"() -> (w328:T2)
            n206 = Index Array(array=w329) -> (element=w332:cluster{string[]})  [unwired: 1 in]
            n207 = Unbundle(w328) -> ("Frame Rate"=w327:i32, "Compression"=w326:i32, "Size"=w330:u16)
            n208 = Unbundle(w332) -> (w331:string[])
            n209 = Index Array(array=w331, index=w330) -> (element=w325:string)
            n210 = call-poly <vilib>:"Write Key.vi"("section"=w336, "value"=w325, "key"="Size", "refnum"=w321) -> ("refnum out"=w338:T13)  [unwired: 2 in, 5 out]
            n211 = call-poly <vilib>:"Write Key.vi"("section"=w336, "value"=w327, "key"="FrameRate", "refnum"=w338) -> ("refnum out"=w337:T13)  [unwired: 1 in, 6 out]
            n212 = local write "DB Camera Config"(w339) -> ()
            n213 = property on="Camera Settings" class="Clust (strict)"("Visible"=w339) -> ()  [unwired: 2 in, 2 out]
            n214 = call-poly <vilib>:"Write Key.vi"("section"=w336, "value"=w326, "key"="Compression", "refnum"=w337) -> ("refnum out"=w323:T13)  [unwired: 1 in, 6 out]
            n215 = call <vilib>:"Close Config Data.vi"("refnum"=w323) -> ("file path"=w324:path)  [unwired: 2 in, 8 out]
            n216 = call <vilib>:"Open Config Data.vi"("configuration file path"=w324) -> ("refnum"=w322:T13)  [unwired: 8 in, 2 out]
          }
          frame True {
            n217 = property on="Camera Settings" class="Clust (strict)"("Visible"=TRUE) -> ()  [unwired: 2 in, 2 out]
          }
        }
      }
      event "Camera Settings": Value Change {
        n218 = event-data() -> ("NewVal"=w353:T2)  [unwired: 1 in]
        n219 = Index Array(array=w349) -> (element=w348:cluster{string[]})  [unwired: 1 in]
        n220 = Unbundle(w353) -> ("Frame Rate"=w344:i32, "Compression"=w343:i32, "Size"=w346:u16)
        n221 = Unbundle(w348) -> (w347:string[])
        n222 = Index Array(array=w347, index=w346) -> (element=w345:string)
        n223 = Format Into String(format string="%s   %dfps   %d%%", w345, w344, w343) -> (resulting string=w350:string)  [unwired: 2 in, 1 out]
        n224 = Build Array(w350) -> (w351:string[])
        n225 = property on="DB Camera Config" class="Bool (strict)"("Strings [4]"=w351) -> ()  [unwired: 2 in, 2 out]
      }
      event "Motor.Enable": Value Change {
        n226 = event-data() -> ("NewVal"=w359:bool)  [unwired: 1 in]
        n227 = Unbundle("Motor") -> ("Value"=w358:dbl)  [unwired: 1 out]
        n228 = Select(t=w358, s=w359, f=0.0) -> (s? t:f=w356:dbl)
        n229 = call <vilib>:"NT Write Number.vi"("Numeric"=w356, "Name"=w355) -> ()  [unwired: 9 in, 1 out]
      }
      event "Test Slider": Value Change {
        n230 = event-data() -> ("NewVal"=w362:dbl)  [unwired: 1 in]
        n231 = call <vilib>:"NT Write Number.vi"("Numeric"=w362, "Name"=w363) -> ()  [unwired: 9 in, 1 out]
      }
      event "On/Off": Value Change {
        n232 = event-data() -> ("NewVal"=w367:bool)  [unwired: 1 in]
        n233 = Boolean To (0,1)(Boolean=w367) -> (0, 1=w366:i16)
        n234 = call <vilib>:"NT Write Number.vi"("Numeric"=w366, "Name"=w365) -> ()  [unwired: 9 in, 1 out]
      }
      event "Rev/Fwd": Value Change {
        n235 = event-data() -> ("NewVal.Forward"=w375:bool, "NewVal.Reverse"=w374:bool)  [unwired: 1 in]
        n236 = Boolean To (0,1)(Boolean=w375) -> (0, 1=w371:i16)
        n237 = Boolean To (0,1)(Boolean=w374) -> (0, 1=w373:i16)
        n238 = Negate(x=w373) -> (-x=w372:i16)
        n239 = Add(x=w371, y=w372) -> (x+y=w370:i16)
        n240 = call <vilib>:"NT Write Number.vi"("Numeric"=w370, "Name"=w369) -> ()  [unwired: 9 in, 1 out]
      }
      event "Test Ring": Value Change {
        n241 = event-data() -> ("NewVal"=w379:u16)  [unwired: 1 in]
        n242 = property on="Test Ring" class="Ring (strict)"() -> ("Strings []"=w380:string[])  [unwired: 2 in, 2 out]
        n243 = Index Array(array=w380, index=w379) -> (element=w378:string)
        n244 = call <vilib>:"NT Write String.vi"("String"=w378, "Name"=w377) -> ()  [unwired: 9 in, 1 out]
      }
      event "Rec Mode": Value Change {
        # "Update globals for recording mode and path to read log from.\nClear when logging and let NetworkTables set path for vision to\nuse."
        n245 = event-data() -> ("NewVal"=w390:enum32{"Stop", "Record", "Playback"})  [unwired: 1 in]
        n246 = global write "WPI_DashboardLogging Global.vi" "Logging Filename"(path "") -> ()
        n247 = global write "WPI_DashboardLogging Global.vi" "Recording"(w390) -> ()
        n248 = case shown="\"Stop\", \"Record\"" w390 {
          tunnel: w389 -> [_ w392 w400]
          tunnel: [_ _ w399] -> w386
          tunnel: [_ _ w398] -> _
          tunnel: w384 -> [_ _ w396]
          tunnel: cluster{i32, i32} {-250, 170} -> [_ _ w395]
          tunnel: [_ _ T15 {"Image Size"=TRUE, "Image Type"=TRUE, "Pixel Value"=TRUE, "ROI Information"=TRUE, "Zoom Factor"=FALSE} ("Image Information Shown:All Elements")] -> w382
          tunnel: [_ _ TRUE ("Zoom Factor")] -> w381
          frame Default {
          }
          frame "Stop", "Record" {
            # "Place Window too"
            n249 = invoke class="VI" method="FP.Close"(reference=w392) -> (reference out=w391:refnum<vi>)  [unwired: 2 in, 2 out]
            n250 = invoke class="VI" method="Abort VI"(reference=w391) -> ()  [unwired: 2 in, 3 out]
          }
          frame "Playback" {
            n251 = call "Open Playback Panel.vi"("Offset"=w395, "DB VI Ref"=w396, "Playback in"=w400) -> ("Playback out"=w397:refnum<vi>)  [unwired: 8 in]
            n252 = register-events(w397) -> (reference out=w399:refnum<event-registration>, error out=w398:errorcluster)  [unwired: 2 in]
          }
        }
        n253 = property on="Camera Image" class="ImageControl"("Image Information Shown"=w382, "Image Information Visible"=w381) -> ()  [unwired: 2 in, 2 out]
        n254 = call <vilib>:"WPI_DashboardNT Log FieldName Cache.vi"("Operation"=enum16{"Lookup/Add", "Index", "Clear"}."Clear") -> ()  [unwired: 8 in, 3 out]
      }
      event Panel Close {
        w401 = enum32{"Stop", "Record", "Playback"}."Stop" ("Rec Mode")
        n255 = event-data() -> ()  [unwired: 1 in, 4 out]
        n256 = local write "Rec Mode"(w401) -> ()
        n257 = global write "WPI_DashboardLogging Global.vi" "Recording"(w401) -> ()
      }
      event Panel Close {
        # "Abort playback window and ourself"
        n258 = event-data() -> ()  [unwired: 1 in, 4 out]
        n259 = invoke class="VI" method="FP.Close"(reference=w406) -> (reference out=w405:refnum<vi>)  [unwired: 2 in, 2 out]
        n260 = invoke class="VI" method="Abort VI"(reference=w405) -> (error out=w404:errorcluster)  [unwired: 2 in, 2 out]
        n261 = invoke class="VI" method="Abort VI"(error in=w404) -> ()  [unwired: 2 in, 3 out]
      }
    }
  }
  n262 = property on="On/Off" class="Bool (strict)"("Visible"=w25) -> ()  [unwired: 2 in, 2 out]
  n263 = property on="Motor" class="Clust (strict)"("Visible"=w25) -> ()  [unwired: 2 in, 2 out]
  n264 = property on="Progress" class="Clust (strict)"("Visible"=w25) -> ()  [unwired: 2 in, 2 out]
  n265 = property on="Test Ring" class="Ring (strict)"("Visible"=w25) -> ()  [unwired: 2 in, 2 out]
  n266 = property on="Rev/Fwd" class="Clust (strict)"("Visible"=w25) -> ()  [unwired: 2 in, 2 out]
  n267 = local write "DB Camera Config"(w25) -> ()
  n268 = property on="Camera Settings" class="Clust (strict)"("Visible"=w25) -> ()  [unwired: 2 in, 2 out]
  n269 = global write "WPI_DashboardLogging Global.vi" "Recording"(w8) -> ()
  n270 = local write "Rec Mode"(w8) -> ()
